vi "Read VISA Resource.vi"(8 "error in (no error)":errorcluster, 11 "MB_Master_Serial in":refnum<class "MB_Master_Serial.lvclass">) -> (0 "error out":errorcluster, 2 "VISA resource out":refnum<visa-resource-name>, 3 "MB_Master_Serial out":refnum<class "MB_Master_Serial.lvclass">)   [LabVIEW 2023, in "Jiaxin_Stepper_Controller.lvlib" / "MB Master.lvlib" / "MB_Master_Serial.lvclass"]
uses:
  MB_Master_Serial.lvclass
  MB_Master_Serial.lvclass/MB_Master_Serial.ctl
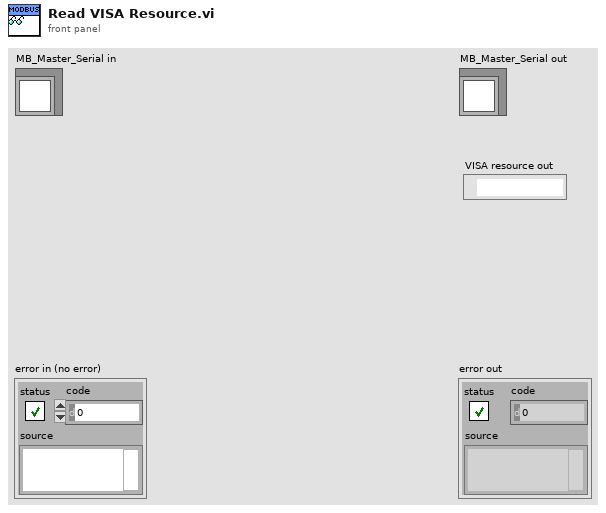
[diagram p1: front panel]
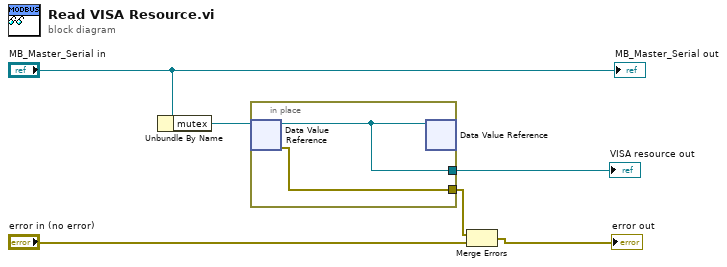
[diagram p0: block diagram]
diagram:
  n1 = Unbundle By Name("MB_Master_Serial in") -> ("mutex"=w2:refnum<data-value>)
  n2 = in-place {
    in-place-border: [w8] -> w1
    in-place-border: [w7] -> w3
    n3 = in-place-dvr #1(w2) -> (w7:refnum<visa-resource-name>, w8:errorcluster)
    n4 = in-place-dvr #1(w7) -> ()  [unwired: 2 out]
  }
  "VISA resource out" <- w3
  n5 = Merge Errors(w1, "error in (no error)") -> (→"error out":errorcluster)
  "MB_Master_Serial out" <- "MB_Master_Serial in"
